vi "ProgramState.vi"(0 "DashboardServer in":refnum<class "Dashboard Server.lvclass">, 5 "error in (no error)":errorcluster) -> (14 "DashboardServer out":refnum<class "Dashboard Server.lvclass">, 15 "programState":string, 19 "error out":errorcluster)   [LabVIEW 2016, in "Dashboard Server.lvclass"]
uses:
  Dashboard Server.lvclass
panel:
  out "returnStatus":string
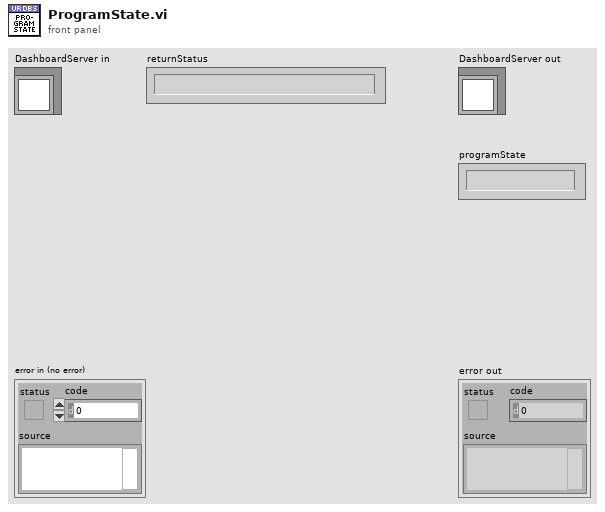
[diagram p1: front panel]
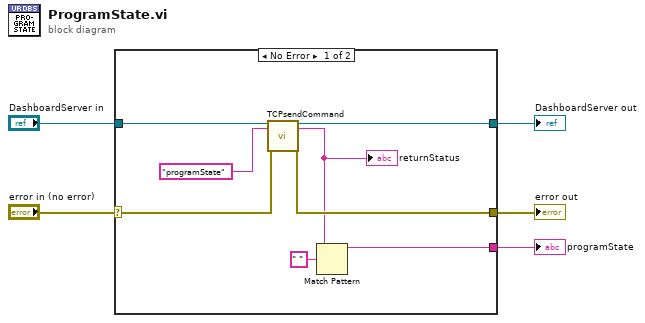
[diagram p0: block diagram]
diagram:
  n1 = case shown="No Error" "error in (no error)" {
    selector: "error in (no error)" -> [w11 w15]
    tunnel: [w10 w15] -> w4
    tunnel: [w12 w14] -> w2
    tunnel: "DashboardServer in" -> [w13 w14]
    tunnel: [w6 _] -> w1
    frame No Error {
      n2 = call-dynamic "TCPsendCommand.vi"("DashboardServer in"=w13, "command"="programState", "error in (no error)"=w11) -> ("DashboardServer out"=w12:refnum<class "Dashboard Server.lvclass">, "returnStatus"=w8:string, "error out"=w10:errorcluster)  [unwired: 13 in, 1 out]
      "returnStatus" <- w8
      n3 = Match Pattern(string=w8, regular expression=" ") -> (before substring=w6:string)  [unwired: 1 in, 3 out]
    }
    frame Error {
    }
  }
  "error out" <- w4
  "DashboardServer out" <- w2
  "programState" <- w1
